vi "MAIN_HGB2_rev02.vi"() -> ()   [LabVIEW 2016]
uses:
  Producer_Case_Structure.ctl
  Consumer Control.ctl
  <vilib>/Utility/error.llb/DialogType.ctl
  <vilib>/DAQmx/write.llb/DAQmx Write (Analog 1D DBL NChan 1Samp).vi
  <vilib>/DAQmx/miscellaneous.llb/DAQmx Fill In Error Info.vi
  <vilib>/express/express analysis/Spectral/Block/exnSpectralBlock spectral measurements RMS poly.vi
  <vilib>/express/express analysis/Spectral/Block/exnSpectralBlock spectral measurements RMS array WFM.vi
  <vilib>/express/express analysis/Spectral/XNode/ExpressSpectralMeasurementsBlockNode.xnode
panel:
  in  "Numeric":i32
  out "Producer":i32=3
  out "Control":i32
  out "On/Off":bool
  in  "On/Off":bool
  in  "Speed Setpoint":dbl=12.0
  in  "Operator Notes":string
  in  "Dummy Variable":dbl
  in  "Record Data":bool
  in  "Sample Rate [S/s]":dbl=10.0
  in  "file path":path=path "S:/002 - Projects/200804 AECSSB/6-Testing/TDMS Data/raw/JunkData/080621-22"
  in  "Stop":bool
  in  "Tab Control":T1(tab)=enum."Pressure & Temperature"
  out "System Temperatures":waveform(dbl)[](graph)=[{"t0"=timestamp(3711052962.8838773 s since 1904-01-01), "dt"=0.1, "Y"=[31.970041267572608, 31.970041267572608, 31.970041267572608, 31.970041267572608, 31.970041267572608], "attributes"=variant("NI_ChannelName"=variant(string "T_dis"), "NI_UnitDescription"=variant(string "Deg C"))}, {"t0"=timestamp(3711052962.8838773 s since 1904-01-01), "dt"=0.1, "Y"=[31.83662326337295, 31.83662326337295, 31.83662326337295, 31.83662326337295, 31.83662326337295], "attributes"=variant("NI_ChannelName"=variant(string "T_liq_mix"), "NI_UnitDescription"=variant(string "Deg C"))}, {"t0"=timestamp(3711052962.8838773 s since 1904-01-01), "dt"=0.1, "Y"=[31.603730023404285, 31.603730023404285, 31.603730023404285, 31.603730023404285, 31.603730023404285], "attributes"=variant("NI_ChannelName"=variant(string "T_gas_mix"), "NI_UnitDescription"=variant(string "Deg C"))}, {"t0"=timestamp(3711052962.8838773 s since 1904-01-01), "dt"=0.1, "Y"=[31.92384492430973, 31.92384492430973, 31.92384492430973, 31.92384492430973, 31.92384492430973], "attributes"=variant("NI_ChannelName"=variant(string "T_wf_cond_out"), "NI_UnitDescription"=variant(string "Deg C"))}, {"t0"=timestamp(3711052962.8838773 s since 1904-01-01), "dt"=0.1, "Y"=[31.708805087588694, 31.708805087588694, 31.708805087588694, 31.708805087588694, 31.708805087588694], "attributes"=variant("NI_ChannelName"=variant(string "T_cf_in"), "NI_UnitDescription"=variant(string "Deg C"))}]
  out "Power Constituents":waveform(dbl)[](graph)=[{"t0"=timestamp(3711052962.8838773 s since 1904-01-01), "dt"=0.1, "Y"=[-0.24580483273071252, -0.24595192787806752, -0.24590289616227778, -0.24565773758337173, -0.24570676929914725], "attributes"=variant("NI_ChannelName"=variant(string "Voltage"))}, {"t0"=timestamp(3711052962.8838773 s since 1904-01-01), "dt"=0.1, "Y"=[-0.03007573285107057, -0.029814230366898897, -0.029846918177419468, -0.029961325514246795, -0.029520040072203102], "attributes"=variant("NI_ChannelName"=variant(string "Frequency"))}, {"t0"=timestamp(3711052962.5858755 s since 1904-01-01), "dt"=0.1, "Y"=[0.0494535006582737, 0.028822120279073715, 0.003032894805073738, 0.013348584994673729, 0.028822120279073715], "attributes"=variant("NI_ChannelName"=variant(string "Torque"))}]
  out "System Pressures":waveform(dbl)[](graph)=[{"t0"=timestamp(3711052962.8838773 s since 1904-01-01), "dt"=0.1, "Y"=[791.0745281409704, 791.0295658631055, 791.154986953992, 791.149239895919, 791.1086724271686], "attributes"=variant("NI_ChannelName"=variant(string "P_comp_suc"))}, {"t0"=timestamp(3711052962.8838773 s since 1904-01-01), "dt"=0.1, "Y"=[791.3763820350057, 791.363873732141, 791.3939612714641, 791.4162733792768, 791.2567080021922], "attributes"=variant("NI_ChannelName"=variant(string "P_comp_dis"))}, {"t0"=timestamp(3711052962.8838773 s since 1904-01-01), "dt"=0.1, "Y"=[791.1641146344607, 791.0407219170118, 791.1025873068561, 791.1752706883669, 791.126251663627], "attributes"=variant("NI_ChannelName"=variant(string "P_comp_int"))}]
  out "Mass Flow":waveform(dbl)(graph)={"t0"=timestamp(3711052962.8838773 s since 1904-01-01), "dt"=0.1, "Y"=[-2.265486306986947e-05, -2.2618089283030912e-05, -2.2630347211977098e-05, -2.2728410643543112e-05, -2.256905756724964e-05], "attributes"=variant("NI_ChannelName"=variant(string "m_dot_wf"))}
  out "Raw Acceleration":waveform(dbl)[](graph)
  out "Accel. Spectrum":cluster{"f0":dbl, "df":dbl, "magnitude":dbl[]}[](graph)
  in  "?":path=path "C:/Users/ASITest/Desktop/REFPROP"
  in  "Working Fluid":string="R134A.FLD"
  in  "Ambient Noise [dB]":dbl=74.0
  # "Stop VI"
  # "Air Squared Hot Gas Bypass Test Stand"
  # "Point to where REFPROP is..."
  # "Registar Index of Calc Characteristics"
  # "INPUT NEEDED"
  # "0 = No\n1 = Yes"
  # "0 = No\n1 = Yes"
  # "UNITS:\nkg/s\nC\nRPM\nkPa\nV\nA"
  # "... where is the sensor in the initialization indexing?"
  # "Must have sound meter set up to manual range:\n1. click 'RNG' button on the meter \n2. the value displayed under 'SPL' on the display is the min of the range\n3. ensure the meter is on 'FAST' mode by clicking 'F/S', 'FAST' will be read on display\n4. use the A/C to select 'A' mode displayed on meter\n5. BEFORE INITIALIZING - set ambient noise level to whatever the sensor measures before running\n* the extech 407730 display frequency is not as high as the display freq here, so peak values\nmay not be seen on the sound meter display."
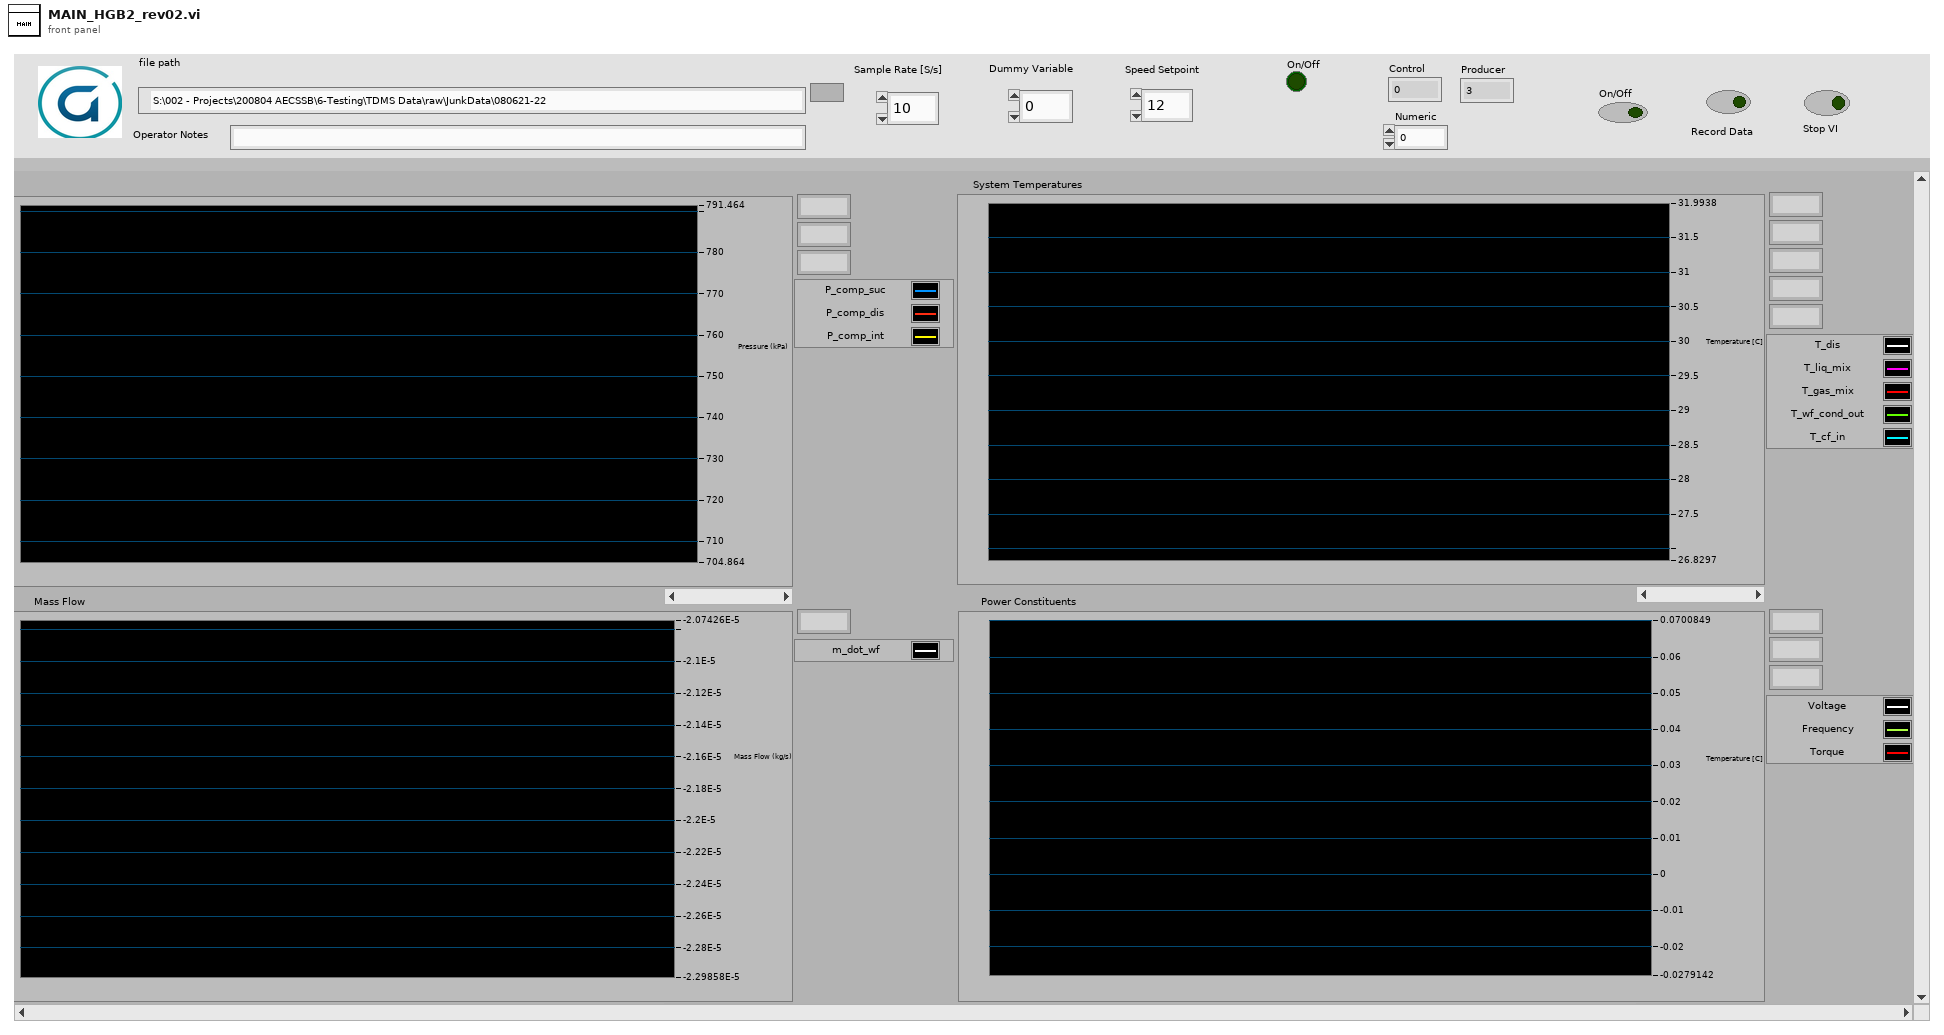
[diagram p1: front panel]
types:
  T1 = enum32{"Schematic", "Pressure & Temperature", "Power", "Acceleration", "Efficiency", "Noise"}
  T2 = typedef "Consumer Control.ctl" = enum16{"System Run", "Shutdown"}
  T3 = enum16{"open", "open or create", "create or replace", "create", "open (read-only)"}
  T4 = typedef "Producer_Case_Structure.ctl" = enum16{"Initialize", "Read", "Write", "Display", "Queue", "Evaluate", "Error"}
  T5 = cluster{"Data Main":waveform(dbl)[], "Accelerometer":waveform(dbl)[], "Dummy Variable":dbl, "Operator Notes":string, "Speed Setpoint":dbl, "NI 6001":waveform(dbl)[], "On/Off":bool}
  T6 = typedef "DialogType.ctl" = u16
  T7 = cluster{"averaging mode":u16, "weighting mode":u16, "number of averages":u32}
  T8 = cluster{"dB On (F)":bool, "unwrap phase (F)":bool, "convert to degree (F)":bool}
  T9 = cluster{"All Channels":tag[], "All Labels":string[], "All Units":string[], "Slope":dbl[], "Y-Intercept":dbl[]}
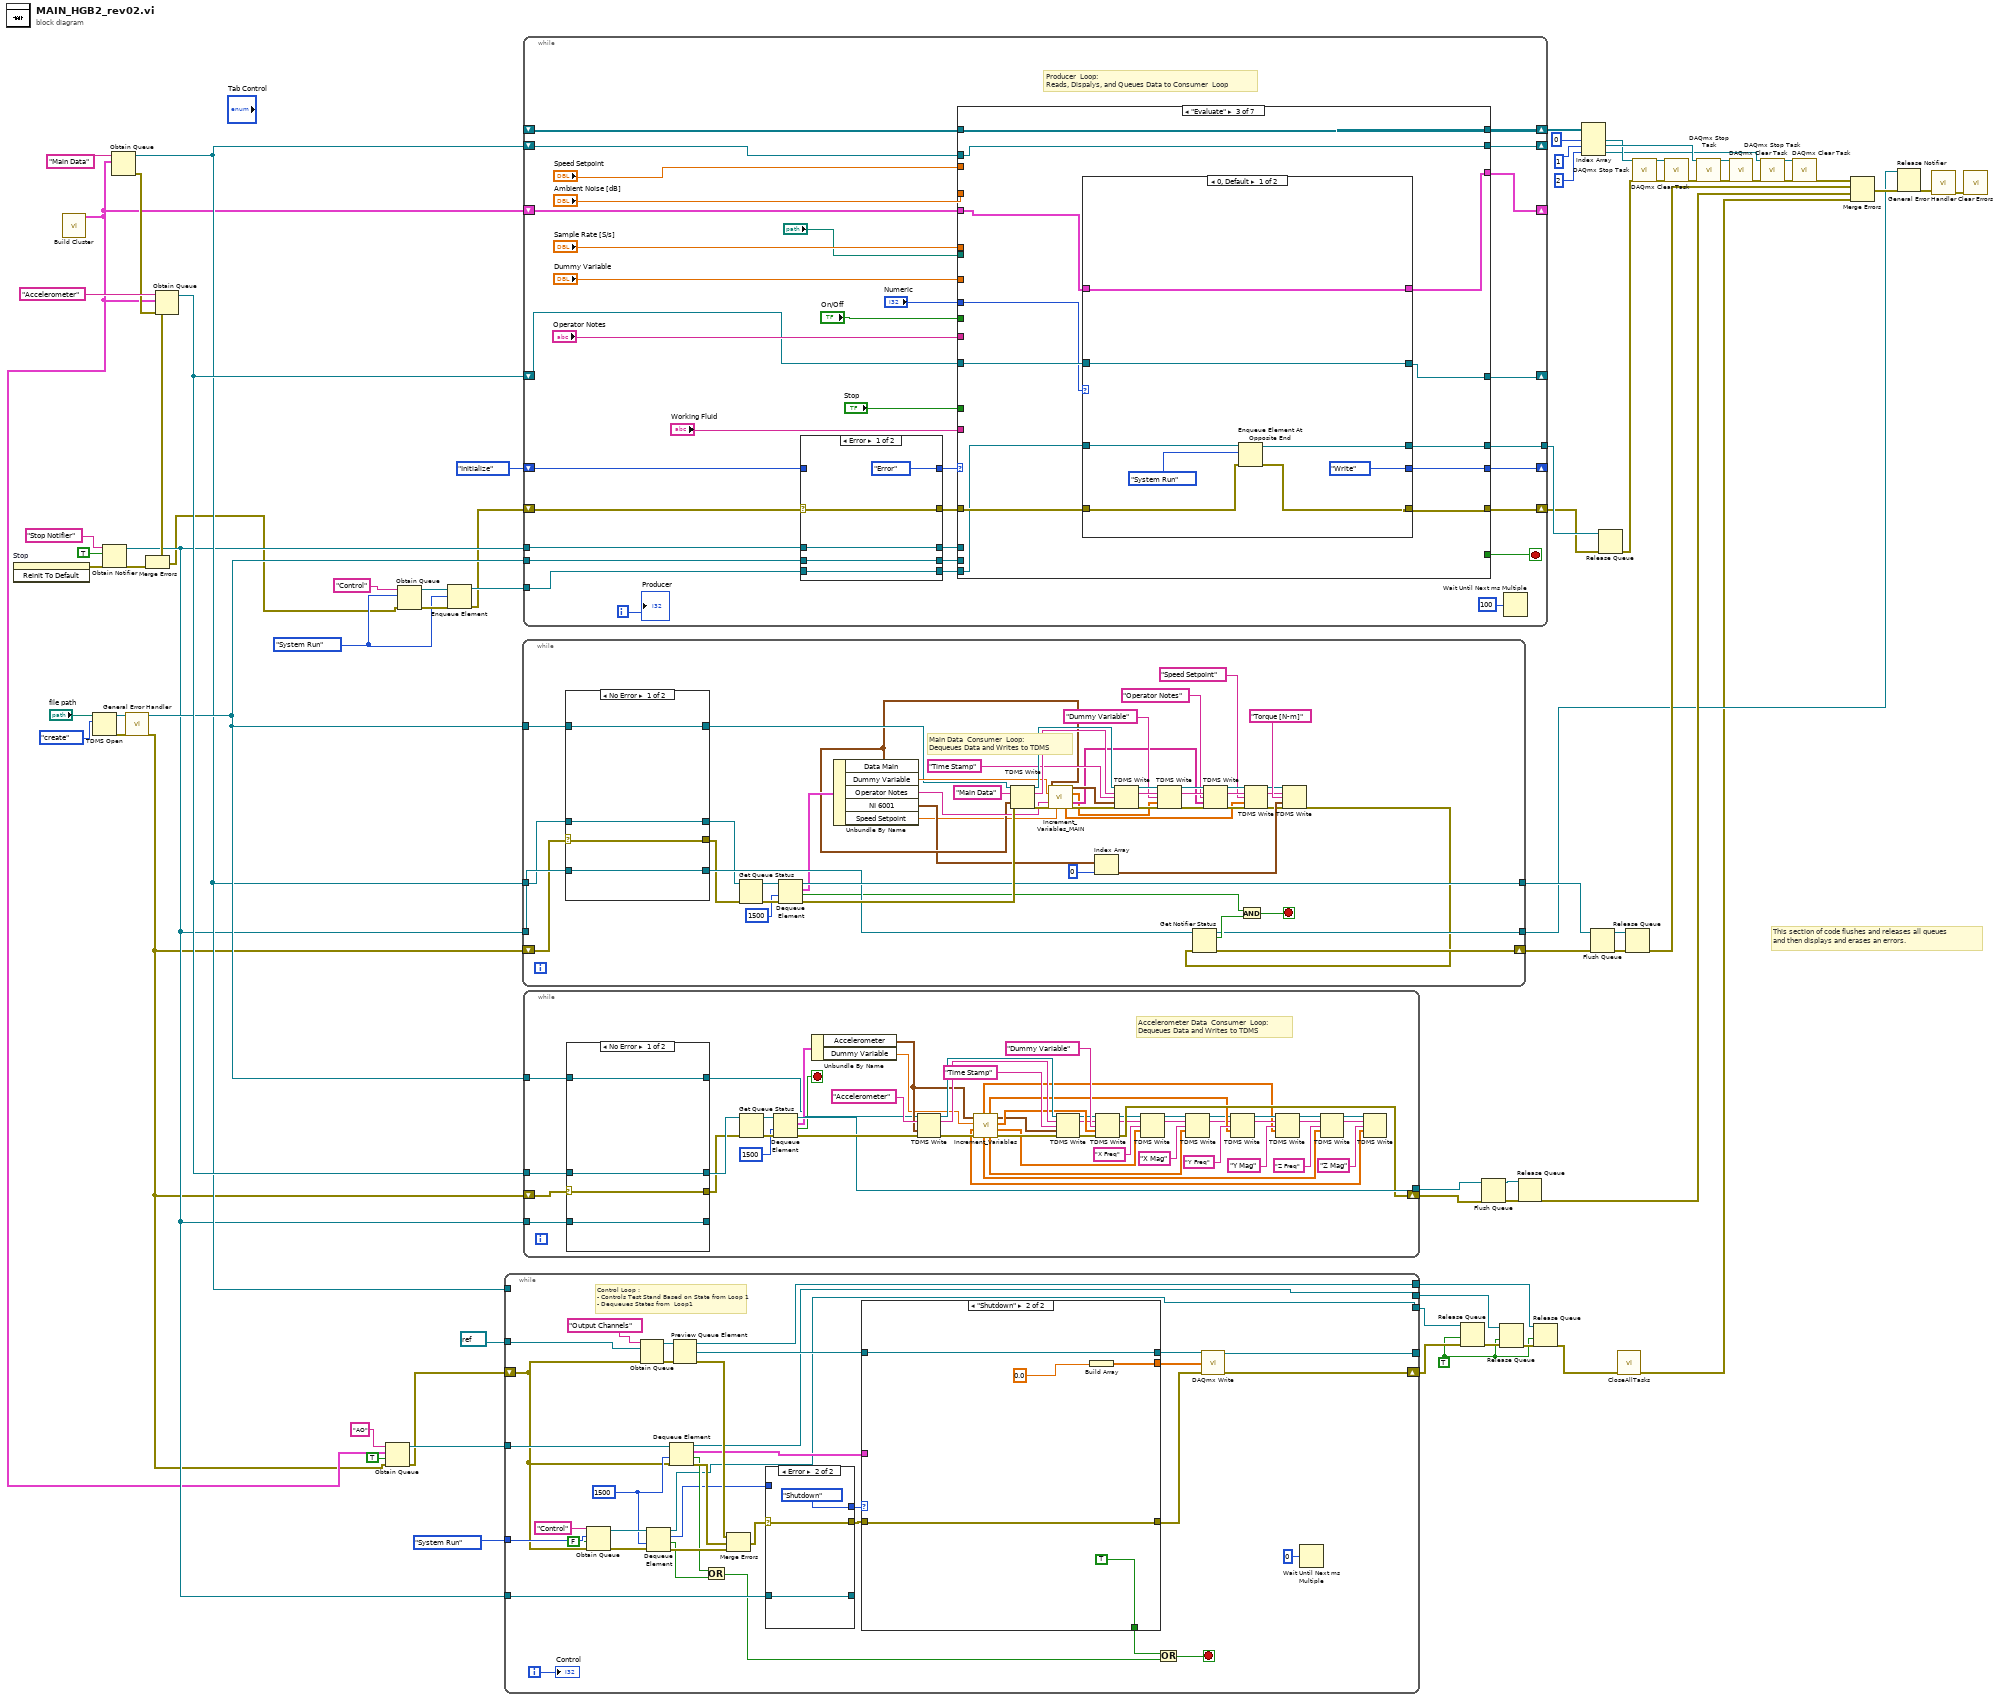
[diagram p0: block diagram]
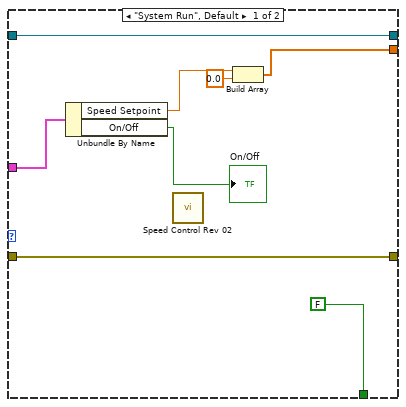
[diagram p3: hidden frame]
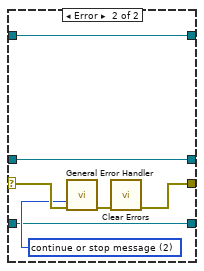
[diagram p4: hidden frame]
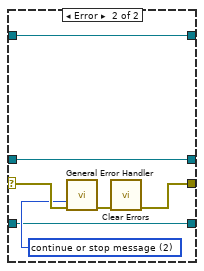
[diagram p5: hidden frame]
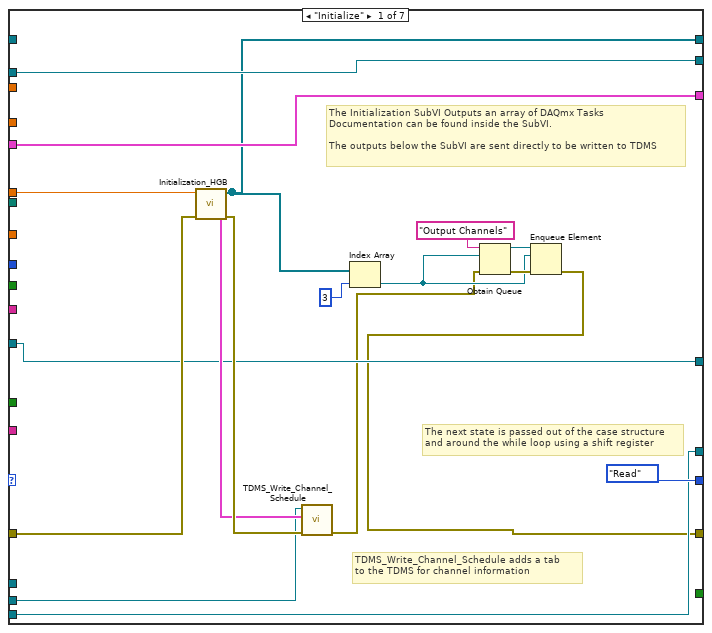
[diagram p6: hidden frame]
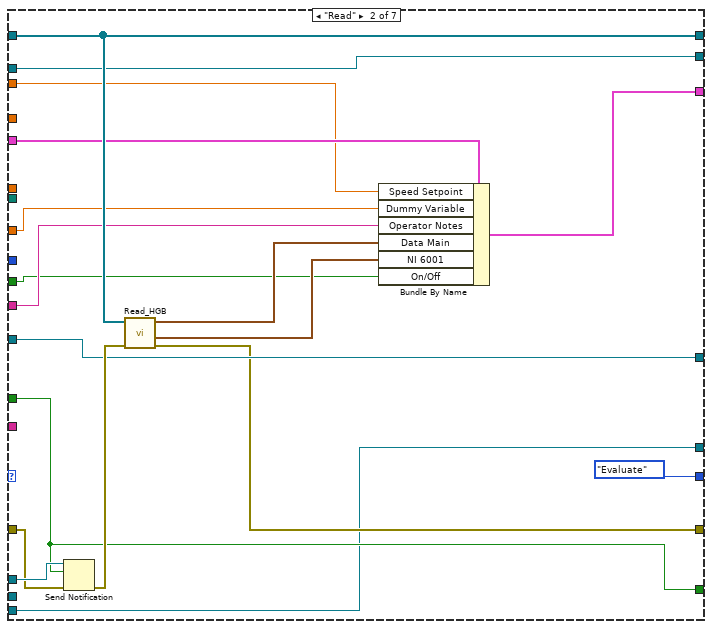
[diagram p7: hidden frame]
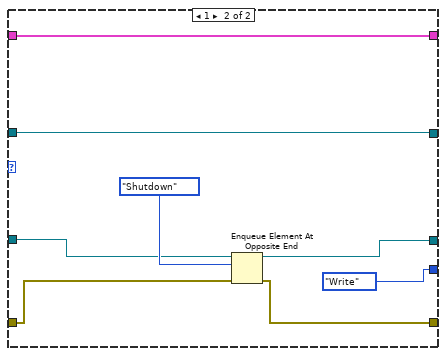
[diagram p8: hidden frame]
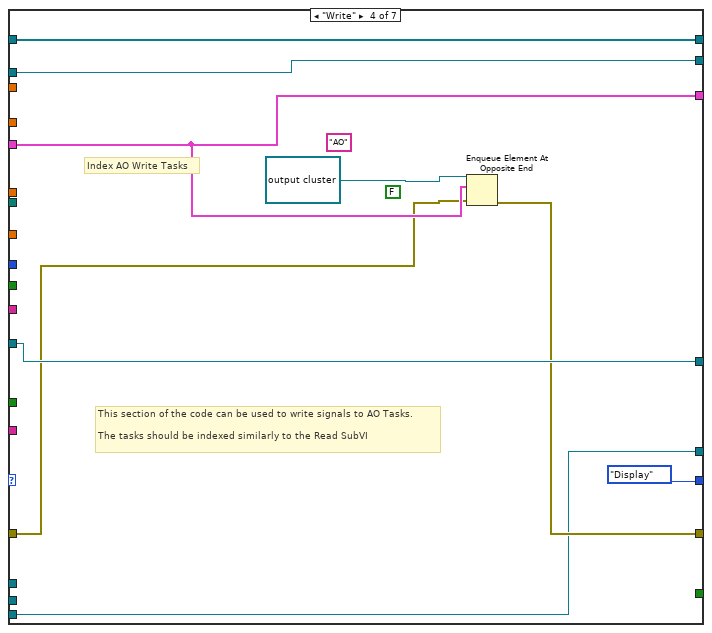
[diagram p9: hidden frame]
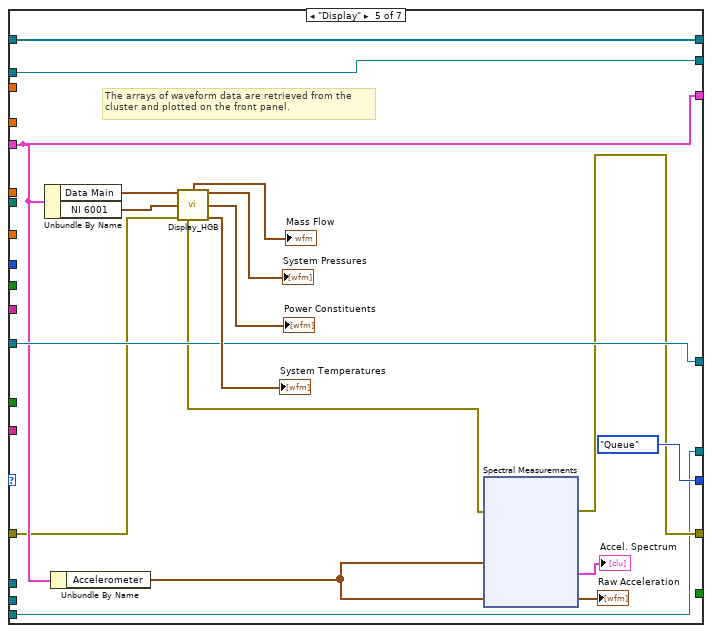
[diagram p10: hidden frame]
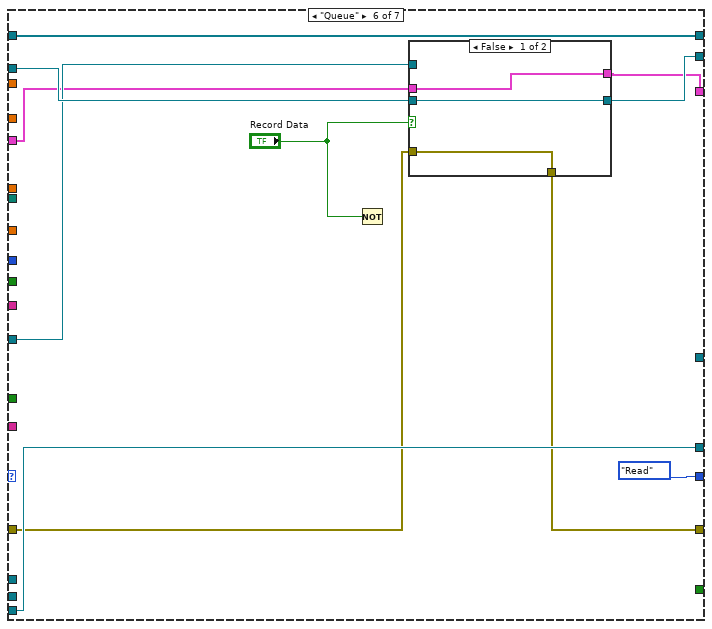
[diagram p11: hidden frame]
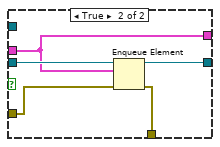
[diagram p12: hidden frame]
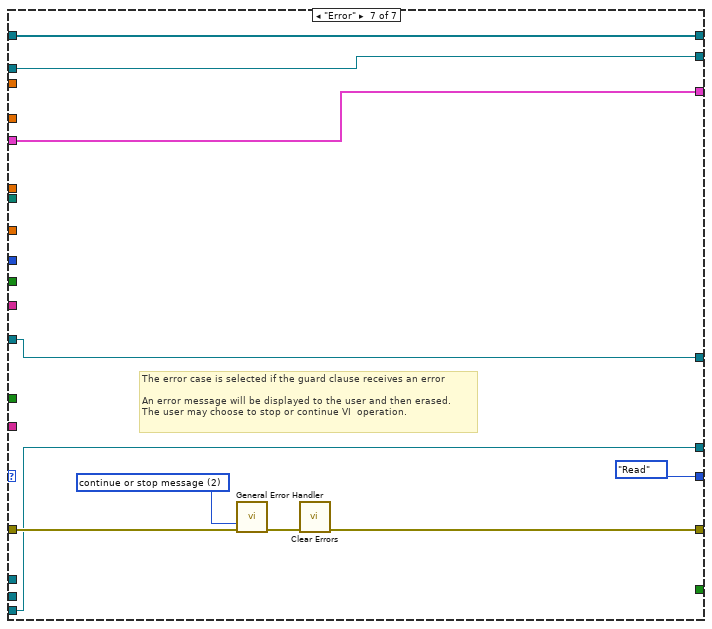
[diagram p13: hidden frame]
diagram:
  w7 = TRUE
  w22 = Consumer_Control."System Run"
  # "This section of code flushes and releases all queues \nand then displays and erases an errors."
  n1 = invoke on="Stop" class="Bool (strict)" method="Reinit To Default"() -> (error out=w68:errorcluster)  [unwired: 3 in, 2 out]
  n2 = call "Build Cluster.vi"() -> ("output cluster"=w3:T5)  [unwired: 11 in]
  n3 = TDMS Open(10:T3."create" ("operation (0:open)"), 11:"file path") -> (0:w63:errorcluster, 3:w44:refnum<k34>)  [unwired: 5 in]
  n4 = Obtain Notifier(name (unnamed)="Stop Notifier", notification data type=TRUE, error in (no error)=w68) -> (notifier out=w31:refnum<notifier>, error out=w61:errorcluster)  [unwired: 1 in, 1 out]
  n5 = Obtain Queue(name (unnamed)="Main Data", element data type=w3) -> (queue out=w36:refnum<queue>, error out=w51:errorcluster)  [unwired: 3 in, 1 out]
  n6 = call <vilib>:"General Error Handler.vi"("error in (no error)"=w63) -> ("error out"=w2:errorcluster)  [unwired: 10 in, 4 out]
  n7 = Obtain Queue(name (unnamed)="Accelerometer", element data type=w3, error in (no error)=w51) -> (queue out=w49:refnum<queue>, error out=w50:errorcluster)  [unwired: 2 in, 1 out]
  n8 = Merge Errors(w50, w61) -> (w17:errorcluster)
  n9 = Obtain Queue(name (unnamed)="AO", element data type=w3, create if not found? (T)=TRUE, error in (no error)=w2) -> (queue out=w4:refnum<queue>, error out=w1:errorcluster)  [unwired: 1 in, 1 out]
  n10 = Obtain Queue(name (unnamed)="Control", element data type=w22, error in (no error)=w17) -> (queue out=w24:refnum<queue>, error out=w23:errorcluster)  [unwired: 2 in, 1 out]
  n11 = Enqueue Element(queue=w24, element=w22, error in (no error)=w23) -> (queue out=w21:refnum<queue>, error out=w16:errorcluster)  [unwired: 1 in, 1 out]
  n12 = while {
    tunnel: [w108] -> _
    shift-right: [w95] -> w15
    shift-left: w1 -> [w74]
    tunnel: refnum<k21> refnum ("task in") -> [w103]
    tunnel: w36 -> [_]
    tunnel: Consumer_Control."System Run" -> [w93]
    tunnel: w31 -> [w87]
    tunnel: [w78] -> w10
    tunnel: [w77] -> w11
    tunnel: [w76] -> w13
    tunnel: w4 -> [w75]
    i -> [w84]
    stop <- w81 stop-if-true
    w98 = 1500 ("timeout in ms (-1)")
    # "Control Loop :\n- Controls Test Stand Based on State from Loop 1\n- Dequeues States from  Loop1"
    n13 = Obtain Queue(name (unnamed)="Control", element data type=w93, create if not found? (T)=FALSE, error in (no error)=w74) -> (queue out=w107:refnum<queue>, error out=w99:errorcluster)  [unwired: 1 in, 1 out]
    n14 = Obtain Queue(name (unnamed)="Output Channels", element data type=w103, error in (no error)=w74) -> (queue out=w104:refnum<queue>, error out=w102:errorcluster)  [unwired: 2 in, 1 out]
    n15 = Dequeue Element(queue=w107, timeout in ms (-1)=w98, error in (no error)=w99) -> (queue out=w76:refnum<queue>, element=w92:T2, timed out?=w96:bool, error out=w100:errorcluster)
    n16 = Dequeue Element(queue=w75, timeout in ms (-1)=w98, error in (no error)=w74) -> (queue out=w77:refnum<queue>, element=w85:T5, timed out?=w97:bool, error out=w101:errorcluster)
    n17 = Preview Queue Element(queue=w104, error in (no error)=w102) -> (queue out=w78:refnum<queue>, element=w105:refnum<k21>, error out=w94:errorcluster)  [unwired: 1 in, 1 out]
    n18 = Or(x=w97, y=w96) -> (x .or. y?=w82:bool)
    n19 = Merge Errors(w94, w101, w100) -> (w91:errorcluster)
    n20 = case shown="Error" w91 {
      selector: w91 -> [w113 w116]
      tunnel: [w113 w116] -> w90
      tunnel: w92 -> [w112 _]
      tunnel: [w112 Consumer_Control."Shutdown"] -> w89
      tunnel: [w111 w115] -> _
      tunnel: w87 -> [w111 w115]
      frame No Error {
      }
      frame Error {
      }
    }
    n21 = case shown="\"Shutdown\"" w89 {
      tunnel: w105 -> [w124 w127]
      tunnel: [w118 w128] -> w110
      tunnel: [w124 w127] -> w109
      tunnel: w85 -> [w121 _]
      tunnel: w90 -> [w122 w125]
      tunnel: [FALSE TRUE] -> w83
      tunnel: [w122 w125] -> w88
      frame "System Run", Default {
        n22 = Unbundle By Name(w121) -> ("Speed Setpoint"=w119:dbl, "On/Off"=→"On/Off":bool)
        n23 = call "Speed Control Rev 02.vi"() -> ()  [unwired: 11 in, 1 out]
        n24 = Build Array(w119, 0.0 ("element")) -> (w118:dbl[])
      }
      frame "Shutdown" {
        n25 = Build Array(0.0 ("Speed Setpoint 2")) -> (w128:dbl[])
      }
    }
    n26 = Or(x=w83, y=w82) -> (x .or. y?=w81:bool)
    n27 = call-poly <vilib>:"DAQmx Write.vi"("task/channels in"=w109, "data"=w110, "error in"=w88) -> ("task out"=w108:refnum<k21>, "error out"=w95:errorcluster)  [unwired: 10 in, 1 out]
    n28 = Wait Until Next ms Multiple(millisecond multiple=u32 0) -> ()  [unwired: 1 out]
    "Control" <- w84
  }
  n29 = while {
    tunnel: w44 -> [w170]
    tunnel: [w180] -> w59
    tunnel: w36 -> [w171]
    tunnel: w31 -> [w173]
    shift-right: [w178] -> w27
    shift-left: w2 -> [w169]
    tunnel: [w148] -> w26
    stop <- w175 stop-if-true
    # "Main Data  Consumer  Loop: \nDequeues Data and Writes to TDMS"
    n30 = case shown="No Error" w169 {
      selector: w169 -> [w186 w192]
      tunnel: [w186 w191] -> w151
      tunnel: w173 -> [w185 w187]
      tunnel: [w185 w187] -> w174
      tunnel: [w184 w189] -> w172
      tunnel: w171 -> [w184 w189]
      tunnel: [w183 w188] -> w149
      tunnel: w170 -> [w183 w188]
      frame No Error {
      }
      frame Error {
        w190 = T6 2 items=["no dialog", "OK message", "continue or stop message", "OK message + warnings", "continue/stop + warnings"] ("type of dialog (OK msg:1)")
        n31 = call <vilib>:"General Error Handler.vi"("type of dialog (OK msg:1)"=w190, "error in (no error)"=w192) -> ("error out"=w193:errorcluster)  [unwired: 9 in, 4 out]
        n32 = call <vilib>:"Clear Errors.vi"("error in (no error)"=w193) -> ("error out"=w191:errorcluster)  [unwired: 5 in, 1 out]
      }
    }
    n33 = Get Queue Status(queue=w172, error in (no error)=w151) -> (queue out=w177:refnum<queue>, error out=w181:errorcluster)  [unwired: 1 in, 6 out]
    n34 = Dequeue Element(queue=w177, timeout in ms (-1)=1500, error in (no error)=w181) -> (queue out=w180:refnum<queue>, element=w150:T5, timed out?=w168:bool, error out=w182:errorcluster)
    n35 = Unbundle By Name(w150) -> ("Data Main"=w140:waveform(dbl)[], "Dummy Variable"=w158:dbl, "Operator Notes"=w146:string, "NI 6001"=w131:waveform(dbl)[], "Speed Setpoint"=w130:dbl)
    n36 = TDMS Write(0:w149, 5:"Main Data" ("group name in (Untitled)"), 9:w140, 11:w182) -> (4:w165:refnum<k34>, 6:w163:string, 15:w166:errorcluster)  [unwired: 2 in, 1 out]
    n37 = call "Increment_Variables_MAIN.vi"("Data Main"=w140, "Dummy Variable"=w158, "Operator Notes"=w146, "error in 2"=w166, "Speed Setpoint"=w130) -> ("Time Stamp"=w159:timestamp[], "Dummy Variable Array"=w133:dbl[], "Operator Notes Array"=w147:string[], "Speed Setpoint Array"=w142:dbl[], "error IO"=w167:errorcluster)  [unwired: 6 in]
    n38 = Index Array(array=w131, index=0) -> (element=w135:waveform(dbl))
    n39 = TDMS Write(0:w165, 5:w163, 7:"Time Stamp" ("group name in (Untitled)"), 9:w159, 11:w167) -> (4:w162:refnum<k34>, 6:w160:string, 15:w161:errorcluster)  [unwired: 1 in, 1 out]
    n40 = TDMS Write(0:w162, 5:w160, 7:"Dummy Variable" ("group name in (Untitled)"), 9:w133, 11:w161) -> (4:w156:refnum<k34>, 6:w155:string, 15:w157:errorcluster)  [unwired: 1 in, 1 out]
    n41 = TDMS Write(0:w156, 5:w155, 7:"Operator Notes" ("group name in (Untitled)"), 9:w147, 11:w157) -> (4:w143:refnum<k34>, 6:w144:string, 15:w145:errorcluster)  [unwired: 1 in, 1 out]
    n42 = TDMS Write(0:w143, 5:w144, 7:"Speed Setpoint" ("group name in (Untitled)"), 9:w142, 11:w145) -> (4:w137:refnum<k34>, 6:w136:string, 15:w134:errorcluster)  [unwired: 1 in, 1 out]
    n43 = TDMS Write(0:w137, 5:w136, 7:"Torque [N-m]" ("channel name(s) in (Untitled)"), 9:w135, 11:w134) -> (15:w132:errorcluster)  [unwired: 1 in, 3 out]
    n44 = Get Notifier Status(notifier=w174, error in (no error)=w132) -> (notifier out=w148:refnum<notifier>, current notification=w179:bool, error out=w178:errorcluster)  [unwired: 2 out]
    n45 = And(x=w168, y=w179) -> (x .and. y?=w175:bool)
  }
  n46 = while {
    shift-right: [w220] -> _
    shift-left: Producer_Case_Structure."Initialize" ("Enum") -> [w226]
    shift-right: [w222] -> w65
    shift-left: _ -> [w221]
    tunnel: w31 -> [w227]
    shift-right: [w217] -> _
    shift-left: w3 -> [w216]
    shift-right: [w214] -> _
    shift-left: w36 -> [w213]
    shift-right: [w223] -> w19
    shift-left: w16 -> [w215]
    tunnel: w44 -> [w208]
    shift-right: [w206] -> _
    shift-left: w49 -> [w207]
    tunnel: w21 -> [w198]
    tunnel: [w196] -> w20
    i -> [w200]
    stop <- w219 stop-if-true
    # "Producer  Loop: \nReads, Dispalys, and Queues Data to Consumer  Loop"
    n47 = case shown="Error" w215 {
      selector: w215 -> [w359 w366]
      tunnel: [w359 w366] -> w224
      tunnel: w227 -> [w361 w365]
      tunnel: [w361 w365] -> w218
      tunnel: w226 -> [_ w364]
      tunnel: [Producer_Case_Structure."Error" ("Enum") w364] -> w225
      tunnel: [w358 w363] -> w209
      tunnel: w208 -> [w358 w363]
      tunnel: w198 -> [w357 w362]
      tunnel: [w357 w362] -> w197
      frame Error {
      }
      frame No Error {
      }
    }
    n48 = case shown="\"Evaluate\"" w225 {
      tunnel: w224 -> [w245 w259 w273 w292 w302 w329 w353]
      tunnel: [w228 w250 w272 w296 w310 w328 w350] -> w223
      tunnel: [w233 w260 w268 w300 w316 w337 w354] -> w222
      tunnel: w221 -> [_ w260 w268 w300 w316 w337 w354]
      tunnel: [Producer_Case_Structure."Read" ("Enum") Producer_Case_Structure."Evaluate" ("Enum") w264 Producer_Case_Structure."Display" ("Enum") Producer_Case_Structure."Queue" ("Enum") Producer_Case_Structure."Read" ("Enum") Producer_Case_Structure."Read" ("Enum")] -> w220
      tunnel: [_ w247 _ _ _ _ _] -> w219
      tunnel: w218 -> [_ w261 _ _ _ _ _]
      tunnel: [w241 w257 w274 w294 w309 w334 w352] -> w217
      tunnel: w216 -> [w241 w253 w275 w294 w309 w332 w352]
      tunnel: [w243 w258 w269 w298 w314 w335 w349] -> w214
      tunnel: w213 -> [w243 w258 w269 w298 w314 w336 w349]
      tunnel: "Sample Rate [S/s]" -> [w242 _ _ _ _ _ _]
      tunnel: "Dummy Variable" -> [_ w254 _ _ _ _ _]
      tunnel: "Operator Notes" -> [_ w256 _ _ _ _ _]
      tunnel: w209 -> [w238 _ _ _ _ _ _]
      tunnel: w207 -> [w237 w255 w267 w297 w312 w333 w348]
      tunnel: [w237 w255 w266 w297 w312 _ w348] -> w206
      tunnel: "Ambient Noise [dB]" -> [_ _ _ _ _ _ _]
      tunnel: "?" -> [_ _ _ _ _ _ _]
      tunnel: "Working Fluid" -> [_ _ _ _ _ _ _]
      tunnel: "Speed Setpoint" -> [_ w251 _ _ _ _ _]
      tunnel: "On/Off" -> [_ w248 _ _ _ _ _]
      tunnel: "Stop" -> [_ w247 _ _ _ _ _]
      tunnel: w197 -> [w230 w246 w271 w295 w301 w330 w347]
      tunnel: [w230 w246 w270 w295 w301 w330 w347] -> w196
      tunnel: "Numeric" -> [_ _ w265 _ _ _ _]
      frame "Initialize" {
        # "TDMS_Write_Channel_Schedule adds a tab \nto the TDMS for channel information"
        # "The next state is passed out of the case structure \nand around the while loop using a shift register"
        # "The Initialization SubVI Outputs an array of DAQmx Tasks\nDocumentation can be found inside the SubVI.\n\nThe outputs below the SubVI are sent directly to be written to TDMS"
        n49 = call "Initialization_HGB.vi"("error in"=w245, "Sample Rate"=w242) -> ("error out"=w240:errorcluster, "Task Array"=w233:refnum<k21>[], "output cluster"=w239:T9)  [unwired: 7 in]
        n50 = call "TDMS_Write_Channel_Schedule.vi"("error in (no error)"=w240, "output cluster"=w239, "Refnum in"=w238) -> ("error out"=w229:errorcluster)  [unwired: 8 in]
        n51 = Index Array(array=w233, index=3) -> (element=w231:refnum<k21>)
        n52 = Obtain Queue(name (unnamed)="Output Channels", element data type=w231, error in (no error)=w229) -> (queue out=w235:refnum<queue>, error out=w234:errorcluster)  [unwired: 2 in, 1 out]
        n53 = Enqueue Element(queue=w235, element=w231, error in (no error)=w234) -> (error out=w228:errorcluster)  [unwired: 1 in, 2 out]
      }
      frame "Read" {
        n54 = Send Notification(notification=w247, notifier=w261, error in (no error)=w259) -> (error out=w263:errorcluster)  [unwired: 1 out]
        n55 = call "Read_HGB.vi"("error in (no error)"=w263, "Task Array"=w260) -> ("error out"=w250:errorcluster, "NI 6001"=w249:waveform(dbl)[], "Data Main"=w252:waveform(dbl)[])  [unwired: 7 in]
        n56 = Bundle By Name(cluster=w253, "Speed Setpoint"=w251, "Dummy Variable"=w254, "Operator Notes"=w256, "Data Main"=w252, "NI 6001"=w249, "On/Off"=w248) -> (w257:T5)
      }
      frame "Evaluate" {
        n57 = case shown="0, Default" w265 {
          tunnel: w275 -> [w283 w291]
          tunnel: [w283 w291] -> w274
          tunnel: w273 -> [w282 w287]
          tunnel: [w281 w286] -> w272
          tunnel: w271 -> [w279 w289]
          tunnel: [w278 w288] -> w270
          tunnel: [w277 w285] -> w266
          tunnel: w267 -> [w277 w285]
          tunnel: [Producer_Case_Structure."Write" ("Enum") Producer_Case_Structure."Write" ("Enum")] -> w264
          frame 0, Default {
            n58 = Enqueue Element At Opposite End(queue=w279, element=Consumer_Control."System Run", error in (no error)=w282) -> (queue out=w278:refnum<queue>, error out=w281:errorcluster)  [unwired: 1 in, 1 out]
          }
          frame 1 {
            n59 = Enqueue Element At Opposite End(queue=w289, element=Consumer_Control."Shutdown", error in (no error)=w287) -> (queue out=w288:refnum<queue>, error out=w286:errorcluster)  [unwired: 1 in, 1 out]
          }
        }
      }
      frame "Write" {
        (unwired) FALSE ("create if not found? (T)")
        (unwired) "AO"
        # "This section of the code can be used to write signals to AO Tasks.\n\nThe tasks should be indexed similarly to the Read SubVI"
        # "Index AO Write Tasks"
        n60 = Enqueue Element At Opposite End(queue=refnum<queue> refnum ("queue out"), element=w294, error in (no error)=w292) -> (error out=w296:errorcluster)  [unwired: 1 in, 2 out]
      }
      frame "Display" {
        # "The arrays of waveform data are retrieved from the \ncluster and plotted on the front panel."
        n61 = Unbundle By Name(w309) -> ("Data Main"=w307:waveform(dbl)[], "NI 6001"=w303:waveform(dbl)[])
        n62 = Unbundle By Name(w309) -> ("Accelerometer"=w308:waveform(dbl)[])
        "Raw Acceleration" <- w308
        n63 = call "Display_HGB.vi"("data"=w307, "NI 6001"=w303, "error in (no error)"=w302) -> ("Mass Flow"=→"Mass Flow":waveform(dbl), "System Pressures"=→"System Pressures":waveform(dbl)[], "Power Constituents"=→"Power Constituents":waveform(dbl)[], "error out"=w311:errorcluster, "System Temperatures"=→"System Temperatures":waveform(dbl)[])  [unwired: 8 in]
        n64 = xnode "Spectral Measurements"("Signals"=w308, "error in (no error)"=w311) -> ("FFT - (RMS)"=→"Accel. Spectrum":cluster{"f0":dbl, "df":dbl, "magnitude":dbl[]}[], "error out"=w310:errorcluster)  [unwired: 1 out]
      }
      frame "Queue" {
        n65 = Not(x="Record Data") -> ()  [unwired: 1 out]
        n66 = case shown="False" "Record Data" {
          tunnel: w332 -> [w340 w344]
          tunnel: w336 -> [w341 w345]
          tunnel: [w341 w346] -> w335
          tunnel: [w340 w344] -> w334
          tunnel: w333 -> [_ _]
          tunnel: w329 -> [w339 w343]
          tunnel: [w339 w342] -> w328
          frame False {
          }
          frame True {
            n67 = Enqueue Element(queue=w345, element=w344, error in (no error)=w343) -> (queue out=w346:refnum<queue>, error out=w342:errorcluster)  [unwired: 1 in, 1 out]
          }
        }
      }
      frame "Error" {
        w355 = T6 2 items=["no dialog", "OK message", "continue or stop message", "OK message + warnings", "continue/stop + warnings"] ("type of dialog (OK msg:1)")
        # "The error case is selected if the guard clause receives an error\n\nAn error message will be displayed to the user and then erased. \nThe user may choose to stop or continue VI  operation."
        n68 = call <vilib>:"General Error Handler.vi"("type of dialog (OK msg:1)"=w355, "error in (no error)"=w353) -> ("error out"=w351:errorcluster)  [unwired: 9 in, 4 out]
        n69 = call <vilib>:"Clear Errors.vi"("error in (no error)"=w351) -> ("error out"=w350:errorcluster)  [unwired: 5 in, 1 out]
      }
    }
    n70 = Wait Until Next ms Multiple(millisecond multiple=u32 100) -> ()  [unwired: 1 out]
    "Producer" <- w200
  }
  n71 = while {
    tunnel: w44 -> [w411]
    tunnel: [w417] -> w46
    tunnel: w49 -> [w412]
    tunnel: w31 -> [w414]
    shift-right: [w392] -> w43
    shift-left: w2 -> [w410]
    stop <- w391 stop-if-true
    # "Accelerometer Data  Consumer  Loop: \nDequeues Data and Writes to TDMS"
    n72 = case shown="No Error" w410 {
      selector: w410 -> [w423 w429]
      tunnel: [w423 w428] -> w402
      tunnel: w414 -> [w422 w424]
      tunnel: [w422 w424] -> _
      tunnel: [w421 w426] -> w413
      tunnel: w412 -> [w421 w426]
      tunnel: [w420 w425] -> w400
      tunnel: w411 -> [w420 w425]
      frame No Error {
      }
      frame Error {
        w427 = T6 2 items=["no dialog", "OK message", "continue or stop message", "OK message + warnings", "continue/stop + warnings"] ("type of dialog (OK msg:1)")
        n73 = call <vilib>:"General Error Handler.vi"("type of dialog (OK msg:1)"=w427, "error in (no error)"=w429) -> ("error out"=w430:errorcluster)  [unwired: 9 in, 4 out]
        n74 = call <vilib>:"Clear Errors.vi"("error in (no error)"=w430) -> ("error out"=w428:errorcluster)  [unwired: 5 in, 1 out]
      }
    }
    n75 = Get Queue Status(queue=w413, error in (no error)=w402) -> (queue out=w416:refnum<queue>, error out=w418:errorcluster)  [unwired: 1 in, 6 out]
    n76 = Dequeue Element(queue=w416, timeout in ms (-1)=1500, error in (no error)=w418) -> (queue out=w417:refnum<queue>, element=w401:T5, timed out?=w391:bool, error out=w419:errorcluster)
    n77 = Unbundle By Name(w401) -> ("Accelerometer"=w404:waveform(dbl)[], "Dummy Variable"=w399:dbl)
    n78 = TDMS Write(0:w400, 5:"Accelerometer" ("group name in (Untitled)"), 9:w404, 11:w419) -> (4:w407:refnum<k34>, 6:w405:string, 15:w408:errorcluster)  [unwired: 2 in, 1 out]
    n79 = call "Increment_Variables.vi"("error in 2"=w408, "Dummy Variable"=w399, "Accelerometer"=w404) -> ("error IO"=w409:errorcluster, "X Accel Freq Array"=w388:dbl[], "Dummy Variable Array"=w397:dbl[], "Time Stamp"=w393:timestamp[], "X Accel Mag Array"=w386:dbl[], "Y Accel Freq Array"=w369:dbl[], "Z Accel Freq Array"=w371:dbl[], "Y Accel Mag Array"=w370:dbl[], "Z Accel Mag Array"=w372:dbl[])
    n80 = TDMS Write(0:w407, 5:w405, 7:"Time Stamp" ("group name in (Untitled)"), 9:w393, 11:w409) -> (4:w394:refnum<k34>, 6:w395:string, 15:w398:errorcluster)  [unwired: 1 in, 1 out]
    n81 = TDMS Write(0:w394, 5:w395, 7:"Dummy Variable" ("group name in (Untitled)"), 9:w397, 11:w398) -> (4:w389:refnum<k34>, 6:w390:string, 15:w392:errorcluster)  [unwired: 1 in, 1 out]
    n82 = TDMS Write(0:w389, 5:w390, 7:"X Freq" ("group name in (Untitled)"), 9:w388) -> (4:w383:refnum<k34>, 6:w384:string)  [unwired: 2 in, 2 out]
    n83 = TDMS Write(0:w383, 5:w384, 7:"X Mag" ("group name in (Untitled)"), 9:w386) -> (4:w368:refnum<k34>, 6:w367:string)  [unwired: 2 in, 2 out]
    n84 = TDMS Write(0:w368, 5:w367, 7:"Y Freq" ("group name in (Untitled)"), 9:w369) -> (4:w380:refnum<k34>, 6:w379:string)  [unwired: 2 in, 2 out]
    n85 = TDMS Write(0:w380, 5:w379, 7:"Y Mag" ("group name in (Untitled)"), 9:w370) -> (4:w381:refnum<k34>, 6:w382:string)  [unwired: 2 in, 2 out]
    n86 = TDMS Write(0:w381, 5:w382, 7:"Z Freq" ("group name in (Untitled)"), 9:w371) -> (4:w378:refnum<k34>, 6:w377:string)  [unwired: 2 in, 2 out]
    n87 = TDMS Write(0:w378, 5:w377, 7:"Z Mag" ("group name in (Untitled)"), 9:w372) -> ()  [unwired: 2 in, 4 out]
  }
  n88 = Release Queue(queue=w13, force destroy? (F)=w7, error in (no error)=w15) -> (error out=w12:errorcluster)  [unwired: 2 out]
  n89 = Flush Queue(queue=w46, error in (no error)=w43) -> (queue out=w48:refnum<queue>, error out=w47:errorcluster)  [unwired: 1 out]
  n90 = Release Queue(queue=w11, force destroy? (F)=w7, error in (no error)=w12) -> (error out=w9:errorcluster)  [unwired: 2 out]
  n91 = Release Queue(queue=w48, error in (no error)=w47) -> (error out=w32:errorcluster)  [unwired: 1 in, 2 out]
  n92 = Release Queue(queue=w10, force destroy? (F)=w7, error in (no error)=w9) -> (error out=w8:errorcluster)  [unwired: 2 out]
  n93 = Index Array(array=w65, index #1=0 ("index"), index #2=1 ("index"), index #3=2 ("index")) -> (element #1=w41:refnum<k21>, element #2=w55:refnum<k21>, element #3=w37:refnum<k21>)
  n94 = Flush Queue(queue=w59, error in (no error)=w27) -> (queue out=w60:refnum<queue>, error out=w58:errorcluster)  [unwired: 1 out]
  n95 = Release Queue(queue=w20, error in (no error)=w19) -> (error out=w18:errorcluster)  [unwired: 1 in, 2 out]
  n96 = call "CloseAllTasks.vi"("error in (no error)"=w8) -> ("error out"=w14:errorcluster)  [unwired: 9 in]
  n97 = Release Queue(queue=w60, error in (no error)=w58) -> (error out=w33:errorcluster)  [unwired: 1 in, 2 out]
  n98 = call <vilib>:"DAQmx Stop Task.vi"("task/channels in"=w41, "error in"=w18) -> ("task out"=w66:refnum<k21>, "error out"=w67:errorcluster)  [unwired: 12 in]
  n99 = call <vilib>:"DAQmx Clear Task.vi"("task in"=w66, "error in"=w67) -> ("error out"=w56:errorcluster)  [unwired: 13 in]
  n100 = call <vilib>:"DAQmx Stop Task.vi"("task/channels in"=w55, "error in"=w56) -> ("task out"=w53:refnum<k21>, "error out"=w57:errorcluster)  [unwired: 12 in]
  n101 = call <vilib>:"DAQmx Clear Task.vi"("task in"=w53, "error in"=w57) -> ("error out"=w38:errorcluster)  [unwired: 13 in]
  n102 = call <vilib>:"DAQmx Stop Task.vi"("task/channels in"=w37, "error in"=w38) -> ("task out"=w39:refnum<k21>, "error out"=w40:errorcluster)  [unwired: 12 in]
  n103 = call <vilib>:"DAQmx Clear Task.vi"("task in"=w39, "error in"=w40) -> ("error out"=w34:errorcluster)  [unwired: 13 in]
  n104 = Merge Errors(w34, w33, w32, w14) -> (w29:errorcluster)
  n105 = Release Notifier(notifier=w26, error in (no error)=w29) -> (error out=w28:errorcluster)  [unwired: 1 in, 2 out]
  n106 = call <vilib>:"General Error Handler.vi"("error in (no error)"=w28) -> ("error out"=w45:errorcluster)  [unwired: 10 in, 4 out]
  n107 = call <vilib>:"Clear Errors.vi"("error in (no error)"=w45) -> ()  [unwired: 5 in, 2 out]
